vi "SMU_Meas and Calculate Resitance_No Publish Data.vi"(7 "Current  Level":dbl=0.01, 8 "error in (no error)":errorcluster, 10 "Pins":string[](array[string]), 11 "Semiconductor Module Context":T1) -> (0 "error Out":errorcluster, 2 "R Array":dbl[](array[numeric]), 3 "Semiconductor Module Context Out":T1)   [LabVIEW 2013]
uses:
  <vilib>/NI_TestStand_SemiconductorModule/NI_TestStand_Semiconductor_Module.lvlibp/PinMap/General/SemiconductorModuleContext.ctl
  <vilib>/NI_TestStand_SemiconductorModule/NI_TestStand_Semiconductor_Module.lvlibp/PinMap/DC Power/PinsToNIDCPowerSessions.vi
  <vilib>/NI_TestStand_SemiconductorModule/NI_TestStand_Semiconductor_Module.lvlibp
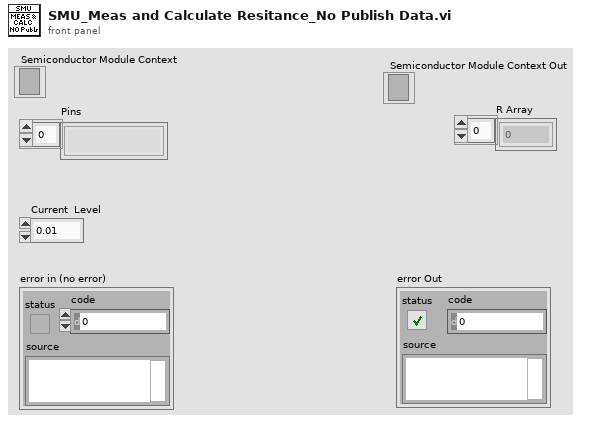
[diagram p1: front panel]
types:
  T1 = typedef "NI_TestStand_Semiconductor_Module.lvlibp/SemiconductorModuleContext.ctl" = refnum<k7>
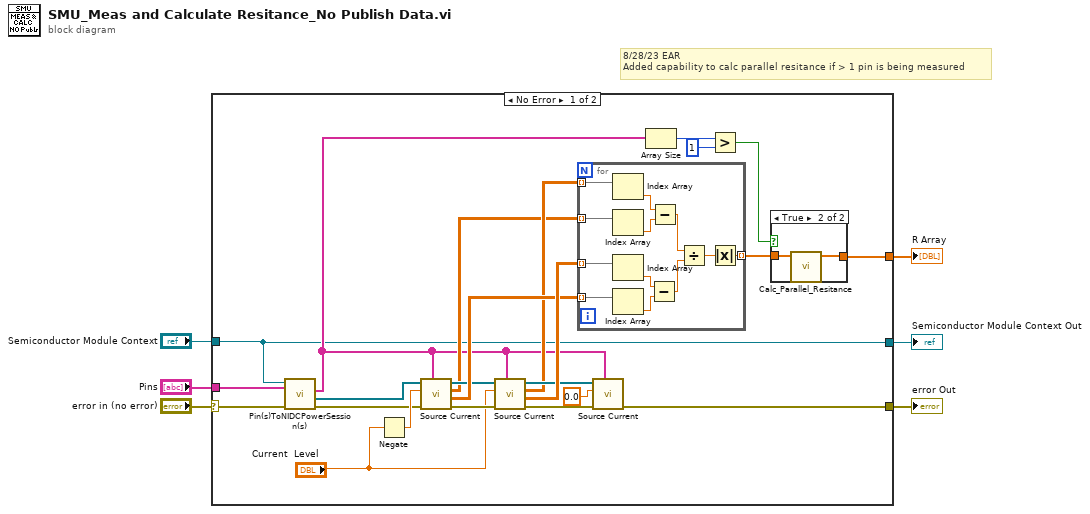
[diagram p0: block diagram]
diagram:
  # "8/28/23 EAR\nAdded capability to calc parallel resitance if > 1 pin is being measured"
  n1 = case shown="No Error" "error in (no error)" {
    selector: "error in (no error)" -> [w29 w46]
    tunnel: "Semiconductor Module Context" -> [w7 w45]
    tunnel: "Pins" -> [w20 _]
    tunnel: [w8 w46] -> w3
    tunnel: [w7 w45] -> w2
    tunnel: [w14 _] -> w1
    frame No Error {
      n2 = call-poly <vilib>:"Pin(s)ToNIDCPowerSession(s).vi"("error in (no error)"=w29, "Pins"=w20, "Semiconductor Module Context"=w7) -> ("error out"=w11:errorcluster, "Instrument Sessions"=w10:refnum<k15>[], "Channel Lists"=w12:string[])  [unwired: 4 in, 2 out]
      n3 = Negate(x="Current  Level") -> (-x=w25:dbl)
      n4 = call "Source Current.vi"("Channel Lists"=w12, "error in (no error)"=w11, "current level"=w25, "Instrument Sessions In"=w10) -> ("error out"=w23:errorcluster, "current measurements"=w27:dbl[][], "voltage measurements"=w21:dbl[][], "Instrument Sessions Out"=w22:refnum<k15>[])  [unwired: 4 in]
      n5 = call "Source Current.vi"("Channel Lists"=w12, "error in (no error)"=w23, "current level"="Current  Level", "Instrument Sessions In"=w22) -> ("error out"=w19:errorcluster, "current measurements"=w28:dbl[][], "voltage measurements"=w24:dbl[][], "Instrument Sessions Out"=w26:refnum<k15>[])  [unwired: 4 in]
      n6 = for {
        tunnel: w24 -> [w36] mode=indexing
        tunnel: w28 -> [w44] mode=indexing
        tunnel: [w42] -> w15 mode=indexing
        tunnel: w27 -> [w40] mode=indexing
        tunnel: w21 -> [w33] mode=indexing
        n7 = Index Array(array=w36) -> (element=w35:dbl)  [unwired: 1 in]
        n8 = Index Array(array=w33) -> (element=w34:dbl)  [unwired: 1 in]
        n9 = Index Array(array=w44) -> (element=w37:dbl)  [unwired: 1 in]
        n10 = Index Array(array=w40) -> (element=w39:dbl)  [unwired: 1 in]
        n11 = Subtract(x=w37, y=w39) -> (x-y=w38:dbl)
        n12 = Subtract(x=w35, y=w34) -> (x-y=w41:dbl)
        n13 = Divide(x=w41, y=w38) -> (x/y=w43:dbl)
        n14 = Absolute Value(x=w43) -> (abs(x)=w42:dbl)
      }
      n15 = call "Source Current.vi"("Channel Lists"=w12, "error in (no error)"=w19, "current level"=0.0, "Instrument Sessions In"=w26) -> ("error out"=w8:errorcluster)  [unwired: 4 in, 3 out]
      n16 = Array Size(array=w12) -> (size(s)=w17:i32)
      n17 = Greater?(x=w17, y=1) -> (0:w13:bool)
      n18 = case shown="True" w13 {
        tunnel: w15 -> [w30 w32]
        tunnel: [w30 w31] -> w14
        frame False {
        }
        frame True {
          n19 = call "Calc_Parallel_Resitance.vi"("Resitance_Per Site"=w32) -> ("Parralel_Resistance"=w31:dbl[])  [unwired: 10 in]
        }
      }
    }
    frame Error {
    }
  }
  "error Out" <- w3
  "Semiconductor Module Context Out" <- w2
  "R Array" <- w1
